vi "svx_SC Line Angle Preprocess.vi"(10 "probe angles Y":u32, 11 "probe angles X":u32) -> (2 "angles Y":dbl, 3 "angles X":dbl, 5 "switch x y axis":bool)   [LabVIEW 2017, in "SVX SC Line.xctl"]
uses:
  <vilib>/addons/_XControls/Shaft Centerline/SVX SC Line.xctl
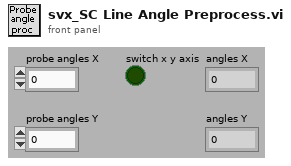
[diagram p1: front panel]
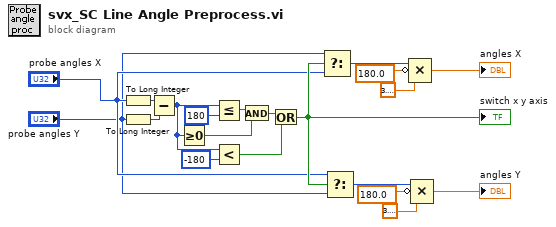
[diagram p0: block diagram]
diagram:
  n1 = To Long Integer(number="probe angles X") -> (32bit integer=w12:i32)
  n2 = To Long Integer(number="probe angles Y") -> (32bit integer=w20:i32)
  n3 = Subtract(x=w12, y=w20) -> (x-y=w16:i32)
  n4 = Greater Or Equal To 0?(x=w16) -> (x >= 0?=w17:bool)
  n5 = Less Or Equal?(x=w16, y=u32 180) -> (x <= y?=w18:bool)
  n6 = Less?(x=w16, y=-180) -> (x < y?=w13:bool)
  n7 = And(x=w18, y=w17) -> (x .and. y?=w14:bool)
  n8 = Or(x=w14, y=w13) -> (x .or. y?=w11:bool)
  "switch x y axis" <- w11
  n9 = Select(t="probe angles Y", s=w11, f="probe angles X") -> (s? t:f=w8:u32)
  n10 = Select(t="probe angles X", s=w11, f="probe angles Y") -> (s? t:f=w5:u32)
  n11 = Compound Arithmetic op=MULTIPLY(w8, invert 180.0 ("value"), 3.141592653589793) -> (→"angles X":dbl)
  n12 = Compound Arithmetic op=MULTIPLY(w5, invert 180.0 ("value"), 3.141592653589793) -> (→"angles Y":dbl)
